vi "IPRegistry.vi"(9 "Action":enum16{"Flush All", "Lookup", "Add"}(ring), 11 "IP Address":string) -> (1 "Users":string[](array[string]), 3 "Success":bool)   [LabVIEW 2013]
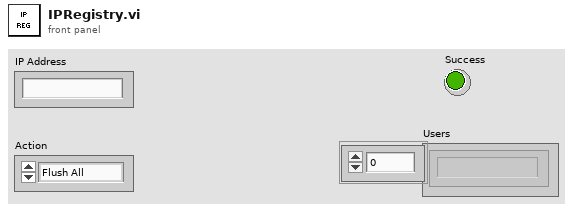
[diagram p1: front panel]
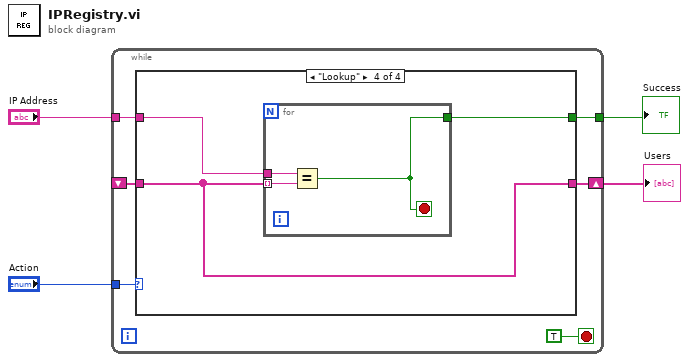
[diagram p0: block diagram]
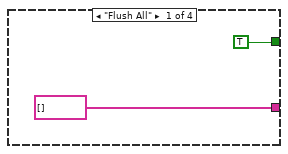
[diagram p2: hidden frame]
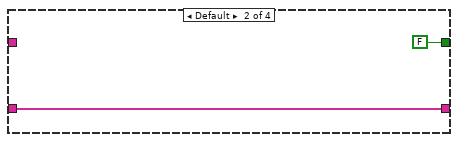
[diagram p3: hidden frame]
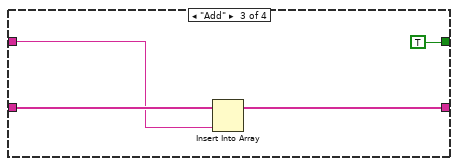
[diagram p4: hidden frame]
diagram:
  n1 = while {
    shift-right: [w7] -> w1
    shift-left: _ -> [w8]
    tunnel: "Action" -> [w9]
    tunnel: [w5] -> w3
    tunnel: "IP Address" -> [w6]
    stop <- TRUE stop-if-true
    n2 = case shown="\"Lookup\"" w9 {
      tunnel: [TRUE FALSE TRUE w19] -> w5
      tunnel: w8 -> [_ w13 w18 w20]
      tunnel: [string[] [] w13 w16 w20] -> w7
      tunnel: w6 -> [_ _ w17 w21]
      frame "Flush All" {
      }
      frame Default {
      }
      frame "Add" {
        n3 = Insert Into Array(array=w18, new element=w17) -> (w16:string[])  [unwired: 1 in]
      }
      frame "Lookup" {
        n4 = for {
          tunnel: w20 -> [w24] mode=indexing
          tunnel: w21 -> [w23]
          tunnel: [w22] -> w19
          stop <- w22 stop-if-true
          n5 = Equal?(x=w23, y=w24) -> (x = y?=w22:bool)
        }
      }
    }
  }
  "Success" <- w3
  "Users" <- w1
